vi "CursorDraw_0_cursorView.vi"(8 "error in (no error)":errorcluster, 11 "Gviewer in":refnum<class "Gviewer.lvclass">) -> (0 "error out":errorcluster, 1 "Focus":i32, 3 "Gviewer out":refnum<class "Gviewer.lvclass">)   [LabVIEW 2020, in "Sgraph_lib_V1.lvlib" / "Gviewer.lvclass"]
doc: "Enable trase selection (s)"
uses:
  Gviewer.lvclass
  Gviewer.lvclass/Gviewer.ctl
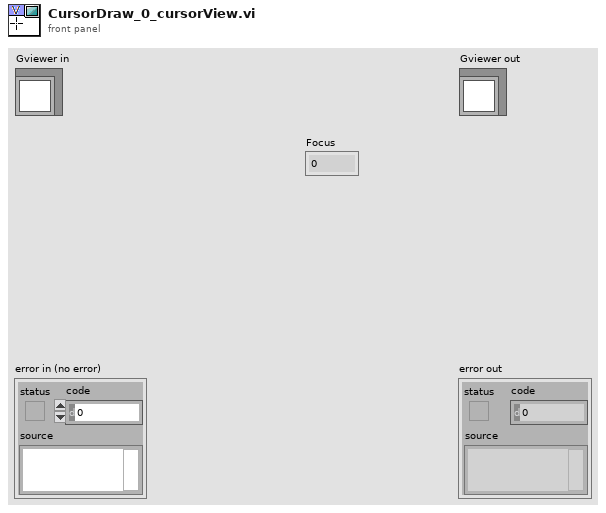
[diagram p1: front panel]
types:
  T1 = typedef "LVPoint32TypeDef.ctl" = cluster{"Horizontal":i32, "Vertical":i32}
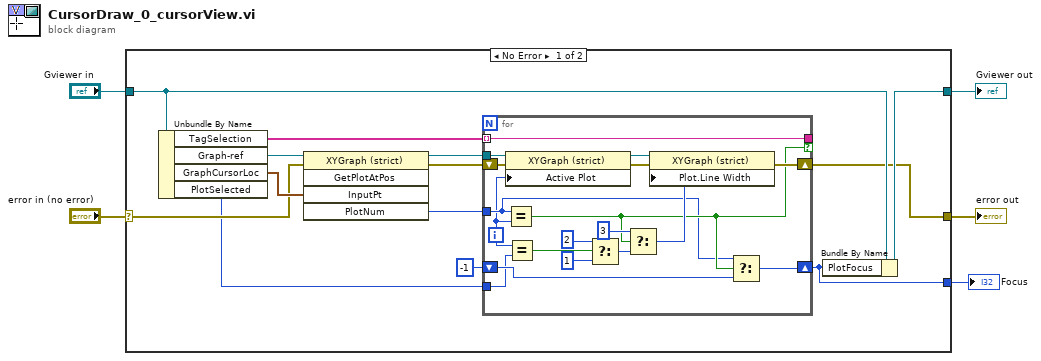
[diagram p0: block diagram]
diagram:
  n1 = case shown="No Error" "error in (no error)" {
    selector: "error in (no error)" -> [w16 w38]
    tunnel: [w7 w38] -> w4
    tunnel: [w8 w37] -> w2
    tunnel: "Gviewer in" -> [w10 w37]
    tunnel: [w6 _] -> w1
    frame No Error {
      n2 = Unbundle By Name(w10) -> ("TagSelection"=w15:string[], "Graph-ref"=w18:refnum<vi>, "GraphCursorLoc"=w17:T1, "PlotSelected"=w9:i32)
      n3 = invoke class="XYGraph (strict)" method="GetPlotAtPos"(reference=w18, error in=w16, "InputPt"=w17) -> (reference out=w13:refnum<vi>, error out=w12:errorcluster, "PlotNum"=w14:i32)  [unwired: 2 in, 2 out]
      n4 = for {
        tunnel: w15 -> [w36] mode=indexing
        tunnel: w14 -> [w25]
        tunnel: [w36] -> _ if=w28
        tunnel: w13 -> [w35]
        shift-right: [w29] -> w7
        shift-left: w12 -> [w31]
        shift-right: [w26] -> w6
        shift-left: -1 -> [w27]
        tunnel: w9 -> [w22]
        i -> [w23]
        n5 = property class="XYGraph (strict)"(reference=w35, error in=w31, "Active Plot"=w23) -> (reference out=w34:refnum<vi>, error out=w30:errorcluster)
        n6 = Equal?(x=w25, y=w23) -> (x = y?=w28:bool)
        n7 = Equal?(x=w23, y=w22) -> (x = y?=w21:bool)
        n8 = Select(t=u8 2 ("Plot.Line Width"), s=w21, f=u8 1 ("Plot.Line Width")) -> (s? t:f=w24:u8)
        n9 = Select(t=u8 3 ("Plot.Line Width"), s=w28, f=w24) -> (s? t:f=w32:u8)
        n10 = property class="XYGraph (strict)"(reference=w34, error in=w30, "Plot.Line Width"=w32) -> (error out=w29:errorcluster)  [unwired: 1 out]
        n11 = Select(t=w25, s=w28, f=w27) -> (s? t:f=w26:i32)
      }
      n12 = Bundle By Name(cluster=w10, "PlotFocus"=w6) -> (w8:refnum<class "Gviewer.lvclass">)
    }
    frame Error {
    }
  }
  "error out" <- w4
  "Gviewer out" <- w2
  "Focus" <- w1
